vi "LNLS Control Decode FOFBC.vi"(8 "error in (no error)":errorcluster, 10 "command body":string) -> (0 "error out":errorcluster, 3 "LNLS Control FOFB Configuration In":T1={"Status"=0, "Operation Mode"=enum."Manual Mode", "Horizontal Gain"=0.0, "Vertical Gain"=0.0, "Selected Reference Orbit"=0, "Selected Correction Matrix"=0, "Selected FPGA Filters"=0, "Horizontal Distortion Threshold"=0.0, "Vertical Distortion Threshold"=0.0, "Fast Command Enabled"=FALSE, "Update Reference Orbit"=FALSE, "Update Contoller Configuration"=FALSE})   [LabVIEW 2011, in "LNLS Control VIs.lvlib"]
uses:
  LNLS Control VIs.lvlib
  Types Definitions/Type Control FOFB Configuration In.ctl
  Types Definitions/Type Operation Mode State.ctl
  Type Definitions.lvlib
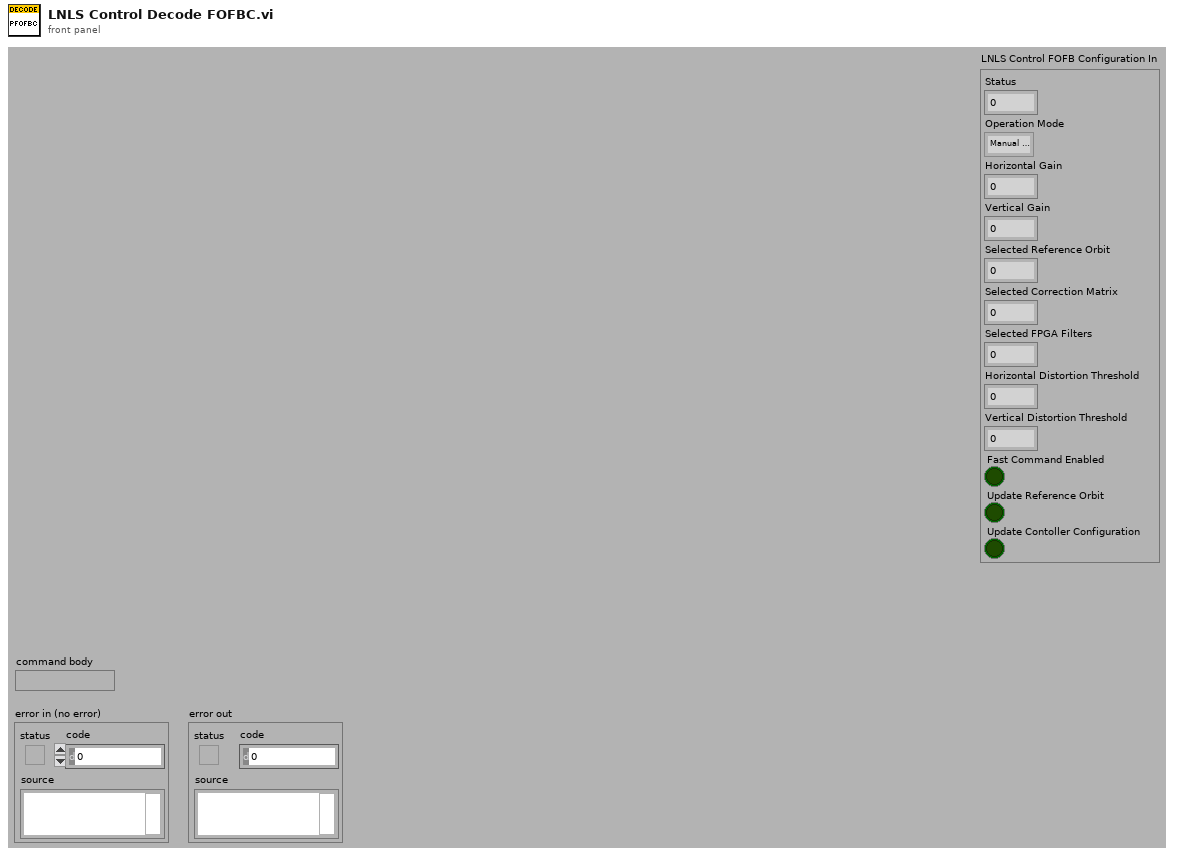
[diagram p1: front panel]
types:
  T1 = typedef "Type Definitions.lvlib/Type Control FOFB Configuration In.ctl" = cluster{"Status":u16, "Operation Mode":T2, "Horizontal Gain":sgl, "Vertical Gain":sgl, "Selected Reference Orbit":i32, "Selected Correction Matrix":i32, "Selected FPGA Filters":i32, "Horizontal Distortion Threshold":sgl, "Vertical Distortion Threshold":sgl, "Fast Command Enabled":bool, "Update Reference Orbit":bool, "Update Contoller Configuration":bool}
  T2 = typedef "Type Definitions.lvlib/Type Operation Mode State.ctl" = enum8{"Idle Mode", "Manual Mode", "FOFB Mode"}
  T3 = enum16{"big-endian, network order", "native, host order", "little-endian"}
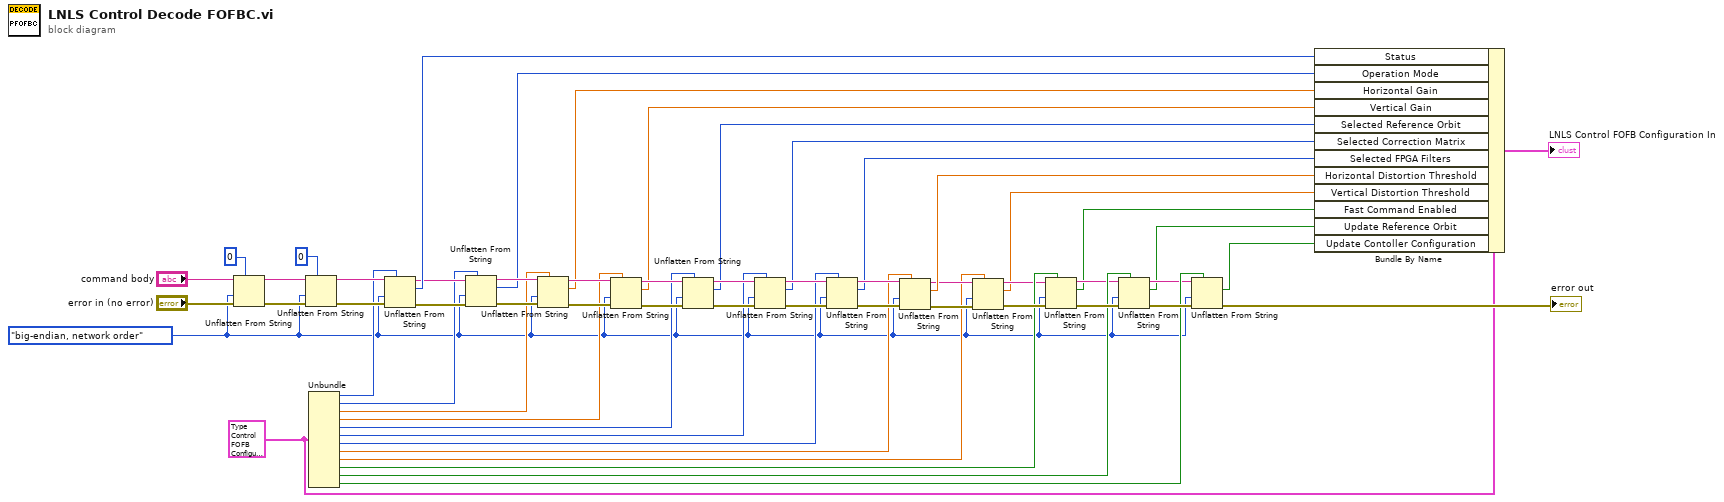
[diagram p0: block diagram]
diagram:
  w11 = T1 {"Status"=0, "Operation Mode"=enum."Idle Mode", "Horizontal Gain"=0.0, "Vertical Gain"=0.0, "Selected Reference Orbit"=0, "Selected Correction Matrix"=0, "Selected FPGA Filters"=0, "Horizontal Distortion Threshold"=0.0, "Vertical Distortion Threshold"=0.0, "Fast Command Enabled"=FALSE, "Update Reference Orbit"=FALSE, "Update Contoller Configuration"=FALSE} ("LNLS Control FOFB Configuration In")
  w1 = T3."big-endian, network order" ("byte order (0:big-endian, network order)")
  n1 = Unflatten From String(type=u8 0 ("priority"), binary string="command body", byte order (0:big-endian, network order)=w1, error in (no error)="error in (no error)") -> (rest of the binary string=w31:string, error out=w55:errorcluster)  [unwired: 1 in, 1 out]
  n2 = Unflatten From String(type=u8 0 ("flag"), binary string=w31, byte order (0:big-endian, network order)=w1, error in (no error)=w55) -> (rest of the binary string=w30:string, error out=w41:errorcluster)  [unwired: 1 in, 1 out]
  n3 = Unbundle(w11) -> ("Status"=w12:u16, "Operation Mode"=w13:T2, "Horizontal Gain"=w14:sgl, "Vertical Gain"=w15:sgl, "Selected Reference Orbit"=w16:i32, "Selected Correction Matrix"=w17:i32, "Selected FPGA Filters"=w18:i32, "Horizontal Distortion Threshold"=w19:sgl, "Vertical Distortion Threshold"=w6:sgl, "Fast Command Enabled"=w20:bool, "Update Reference Orbit"=w21:bool, "Update Contoller Configuration"=w22:bool)
  n4 = Unflatten From String(type=w12, binary string=w30, byte order (0:big-endian, network order)=w1, error in (no error)=w41) -> (rest of the binary string=w29:string, value=w39:u16, error out=w40:errorcluster)  [unwired: 1 in]
  n5 = Unflatten From String(type=w13, binary string=w29, byte order (0:big-endian, network order)=w1, error in (no error)=w40) -> (rest of the binary string=w47:string, value=w38:T2, error out=w52:errorcluster)  [unwired: 1 in]
  n6 = Unflatten From String(type=w14, binary string=w47, byte order (0:big-endian, network order)=w1, error in (no error)=w52) -> (rest of the binary string=w46:string, value=w32:sgl, error out=w51:errorcluster)  [unwired: 1 in]
  n7 = Unflatten From String(type=w15, binary string=w46, byte order (0:big-endian, network order)=w1, error in (no error)=w51) -> (rest of the binary string=w45:string, value=w37:sgl, error out=w53:errorcluster)  [unwired: 1 in]
  n8 = Unflatten From String(type=w16, binary string=w45, byte order (0:big-endian, network order)=w1, error in (no error)=w53) -> (rest of the binary string=w44:string, value=w36:i32, error out=w50:errorcluster)  [unwired: 1 in]
  n9 = Unflatten From String(type=w17, binary string=w44, byte order (0:big-endian, network order)=w1, error in (no error)=w50) -> (rest of the binary string=w43:string, value=w35:i32, error out=w49:errorcluster)  [unwired: 1 in]
  n10 = Unflatten From String(type=w18, binary string=w43, byte order (0:big-endian, network order)=w1, error in (no error)=w49) -> (rest of the binary string=w42:string, value=w34:i32, error out=w48:errorcluster)  [unwired: 1 in]
  n11 = Unflatten From String(type=w19, binary string=w42, byte order (0:big-endian, network order)=w1, error in (no error)=w48) -> (rest of the binary string=w10:string, value=w33:sgl, error out=w26:errorcluster)  [unwired: 1 in]
  n12 = Unflatten From String(type=w6, binary string=w10, byte order (0:big-endian, network order)=w1, error in (no error)=w26) -> (rest of the binary string=w9:string, value=w5:sgl, error out=w25:errorcluster)  [unwired: 1 in]
  n13 = Unflatten From String(type=w20, binary string=w9, byte order (0:big-endian, network order)=w1, error in (no error)=w25) -> (rest of the binary string=w8:string, value=w4:bool, error out=w24:errorcluster)  [unwired: 1 in]
  n14 = Unflatten From String(type=w21, binary string=w8, byte order (0:big-endian, network order)=w1, error in (no error)=w24) -> (rest of the binary string=w7:string, value=w3:bool, error out=w23:errorcluster)  [unwired: 1 in]
  n15 = Unflatten From String(type=w22, binary string=w7, byte order (0:big-endian, network order)=w1, error in (no error)=w23) -> (value=w2:bool, error out=→"error out":errorcluster)  [unwired: 1 in, 1 out]
  n16 = Bundle By Name(cluster=w11, "Status"=w39, "Operation Mode"=w38, "Horizontal Gain"=w32, "Vertical Gain"=w37, "Selected Reference Orbit"=w36, "Selected Correction Matrix"=w35, "Selected FPGA Filters"=w34, "Horizontal Distortion Threshold"=w33, "Vertical Distortion Threshold"=w5, "Fast Command Enabled"=w4, "Update Reference Orbit"=w3, "Update Contoller Configuration"=w2) -> (→"LNLS Control FOFB Configuration In":T1)
